vi "Get Color Transform Matrix.vi"(8 "error in (no error)":errorcluster, 10 "index":i32, 11 "ColorProcessor reference in":refnum<k24>) -> (0 "error out":errorcluster, 2 "GetColorTransformMatrix":sgl[](array[numeric]), 3 "ColorProcessor reference out":refnum<k24>)   [LabVIEW 2015]
uses:
  C:/code/Host/Installer/Scientific Camera Interfaces/LabVIEW/64_bit/Library_X64/Thorlabs.TSI.ColorInterfaces.dll
  64_bit/Library_X64/Thorlabs.TSI.ColorInterfaces.dll
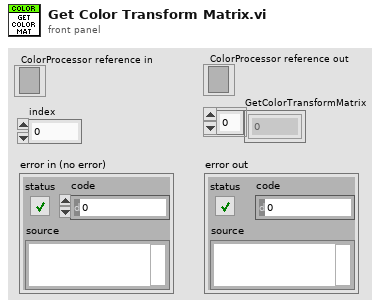
[diagram p1: front panel]
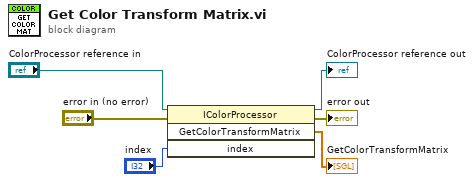
[diagram p0: block diagram]
diagram:
  n1 = invoke class="IColorProcessor" method="GetColorTransformMatrix"(reference="ColorProcessor reference in", error in="error in (no error)", "index"="index") -> (reference out=→"ColorProcessor reference out":refnum<k24>, error out=→"error out":errorcluster, "GetColorTransformMatrix"=→"GetColorTransformMatrix":sgl[])  [unwired: 1 in, 1 out]
